vi "APS set position f.vi"(8 "error in (no error)":errorcluster caption="错误输入（无错误）", 10 "Position":dbl, 11 "Axis_ID":i32) -> (0 "error out":errorcluster caption="错误输出", 3 "function return":i32)   [LabVIEW 2017, in "APS168.lvlib"]
doc: "I32 FNTYPE APS_set_position_f(I32 Axis_ID, F64 Position);"
uses:
  APS168.lvlib
  APS168.dll
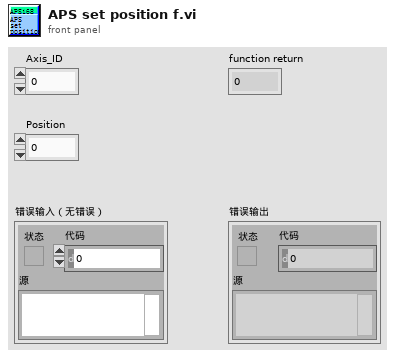
[diagram p1: front panel]
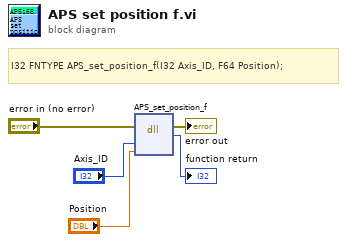
[diagram p0: block diagram]
diagram:
  # "I32 FNTYPE APS_set_position_f(I32 Axis_ID, F64 Position);"
  n1 = dll-call lib="APS168.*" fn="APS_set_position_f"(error in="error in (no error)", "Axis_ID"="Axis_ID", "Position"="Position") -> (error out=→"error out":errorcluster, →"function return":i32)  [unwired: 4 in, 1 out]
